vi "pigeon_ver4_1.vi"() -> ()   [LabVIEW 2015]
uses:
  <vilib>/Platform/TimedLoop/XDataNode/timing_clust.ctl
  <vilib>/Platform/TimedLoop/XDataNode/nitl_modes.ctl
  <vilib>/Platform/TimedLoop/XDataNode/wakeup.ctl
  <vilib>/rvi/Emulation/niFpgaGetClockAttributes.vi
  <vilib>/rvi/Emulation/niFpgaSctlEmulationGetInTimedLoop.vi
  <vilib>/rvi/Emulation/niFpgaEmulationReportErrorSimple.vi
  <vilib>/rvi/eio/common/nirviEmuTemplateMethod_errors.vi
  <vilib>/rvi/Emulation/niFpgaProcessEmulError.vi
  <vilib>/rvi/Emulation/niFpgaCriticalErrorInLSC.vi
  <vilib>/rvi/Memory/Memory_Emulation/nirvimemoryFastEmulation.vi
  <vilib>/rvi/Memory/Memory_Emulation/nirvimemoryEmulation.vi
  <vilib>/rvi/Emulation/niFpgaEmulationIsFPGAContextNoSignature.vi
  <vilib>/rvi/DataTransferAndStorage/Container/Common/niFpgaContainerGetUniqueNameForEmu.vi
  <vilib>/rvi/errors/nirviReportUnexpectedCaseInternalError (U32).vi
  <vilib>/rvi/interface/RandomDataEmulation/niFpgaRandomDataHandleErrors.vi
  <vilib>/eio/EIONode/EIONode.xnode
  <vilib>/Platform/TimedLoop/XDataNode/XDataNode.xnode
  <vilib>/rvi/DataTransferAndStorage/Container/XNode/niFpgaContainer.xnode
  <vilib>/rvi/interface/RandomDataEmulation/nirviRandomDataFpgaReadWriteTemplate.vi
  <vilib>/Platform/TimedLoop/XDataNode/XDNodeRunTimeDep.lvlib
panel:
  in  "AO5":i16
  out "AI2":i16
  in  "Tab Control":enum32{"pigeon"}(tab)
  out "FIFO size":i16
  in  "AO0":i16
  in  "AO1":i16
  in  "AO2":i16
  in  "Run program":bool
  in  "halt processor":bool
  out "control flags":i8 format="%b"
  in  "host operation":i16
  in  "address":u16
  in  "data1":u16
  in  "data2":i32
  in  "repeat program":i32
  out "IP address":i16
  out "PMT1":i16=-4740
  out "ReA":i32
  out "RegB":i16
  out "RegC":i16
  out "exttrigger":bool=TRUE
  out "AI1":i16=161
  out "RegD":i16
  in  "AO4":i16
  in  "AO3":i16
  out "IntTrigger":bool
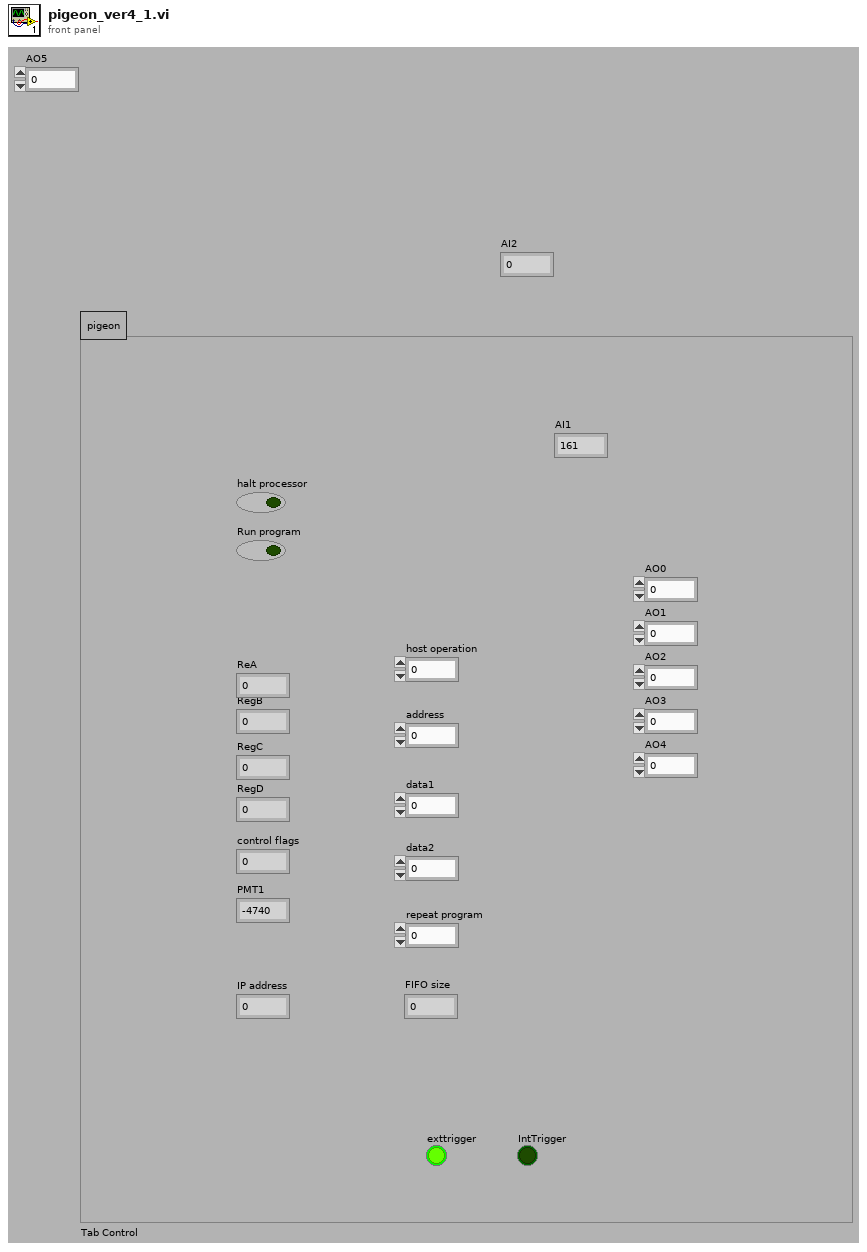
[diagram p1: front panel]
types:
  T1 = typedef "XDNodeRunTimeDep.lvlib/timing_clust.ctl" = cluster{"Expected End [f-1]":u64, "Actual End [f-1]":u64, "Finished Late? [f-1]":bool, "Expected End [i-1]":u64, "Actual End [i-1]":u64, "Finished Late? [i-1]":bool, "Expected Start [i]":u64, "Actual Start [i]":u64, "Expected Start [f]":u64, "Actual Start [f]":u64, "Source Name":string, "Structure Name":string, "Period":i64, "Deadline":i64, "Offset":i64, "Start":i64, "Priority":i32, "Timeout":i32, "Mode":T2, "Wakeup Reason":T3, "Error":errorcluster, "Source Type":string, "Secondary Source Type":string, "Global End Time":u64, "Global Start Time":u64, "Frame Duration":u64, "Iteration Duration":u64, "Assigned CPU":i32, "I/O Scan Engine Mode":u32}
  T2 = typedef "XDNodeRunTimeDep.lvlib/nitl_modes.ctl" = enum32{"No Change", "Process missed periods, maintain original phase", "Discard missed periods, maintain original phase", "Process missed periods, ignore original phase", "Discard missed periods, ignore original phase"}
  T3 = typedef "XDNodeRunTimeDep.lvlib/wakeup.ctl" = enum32{"Normal", "Aborted", "Asynchronous wakeup", "Timing source error", "Timed loop error", "Timeout"}
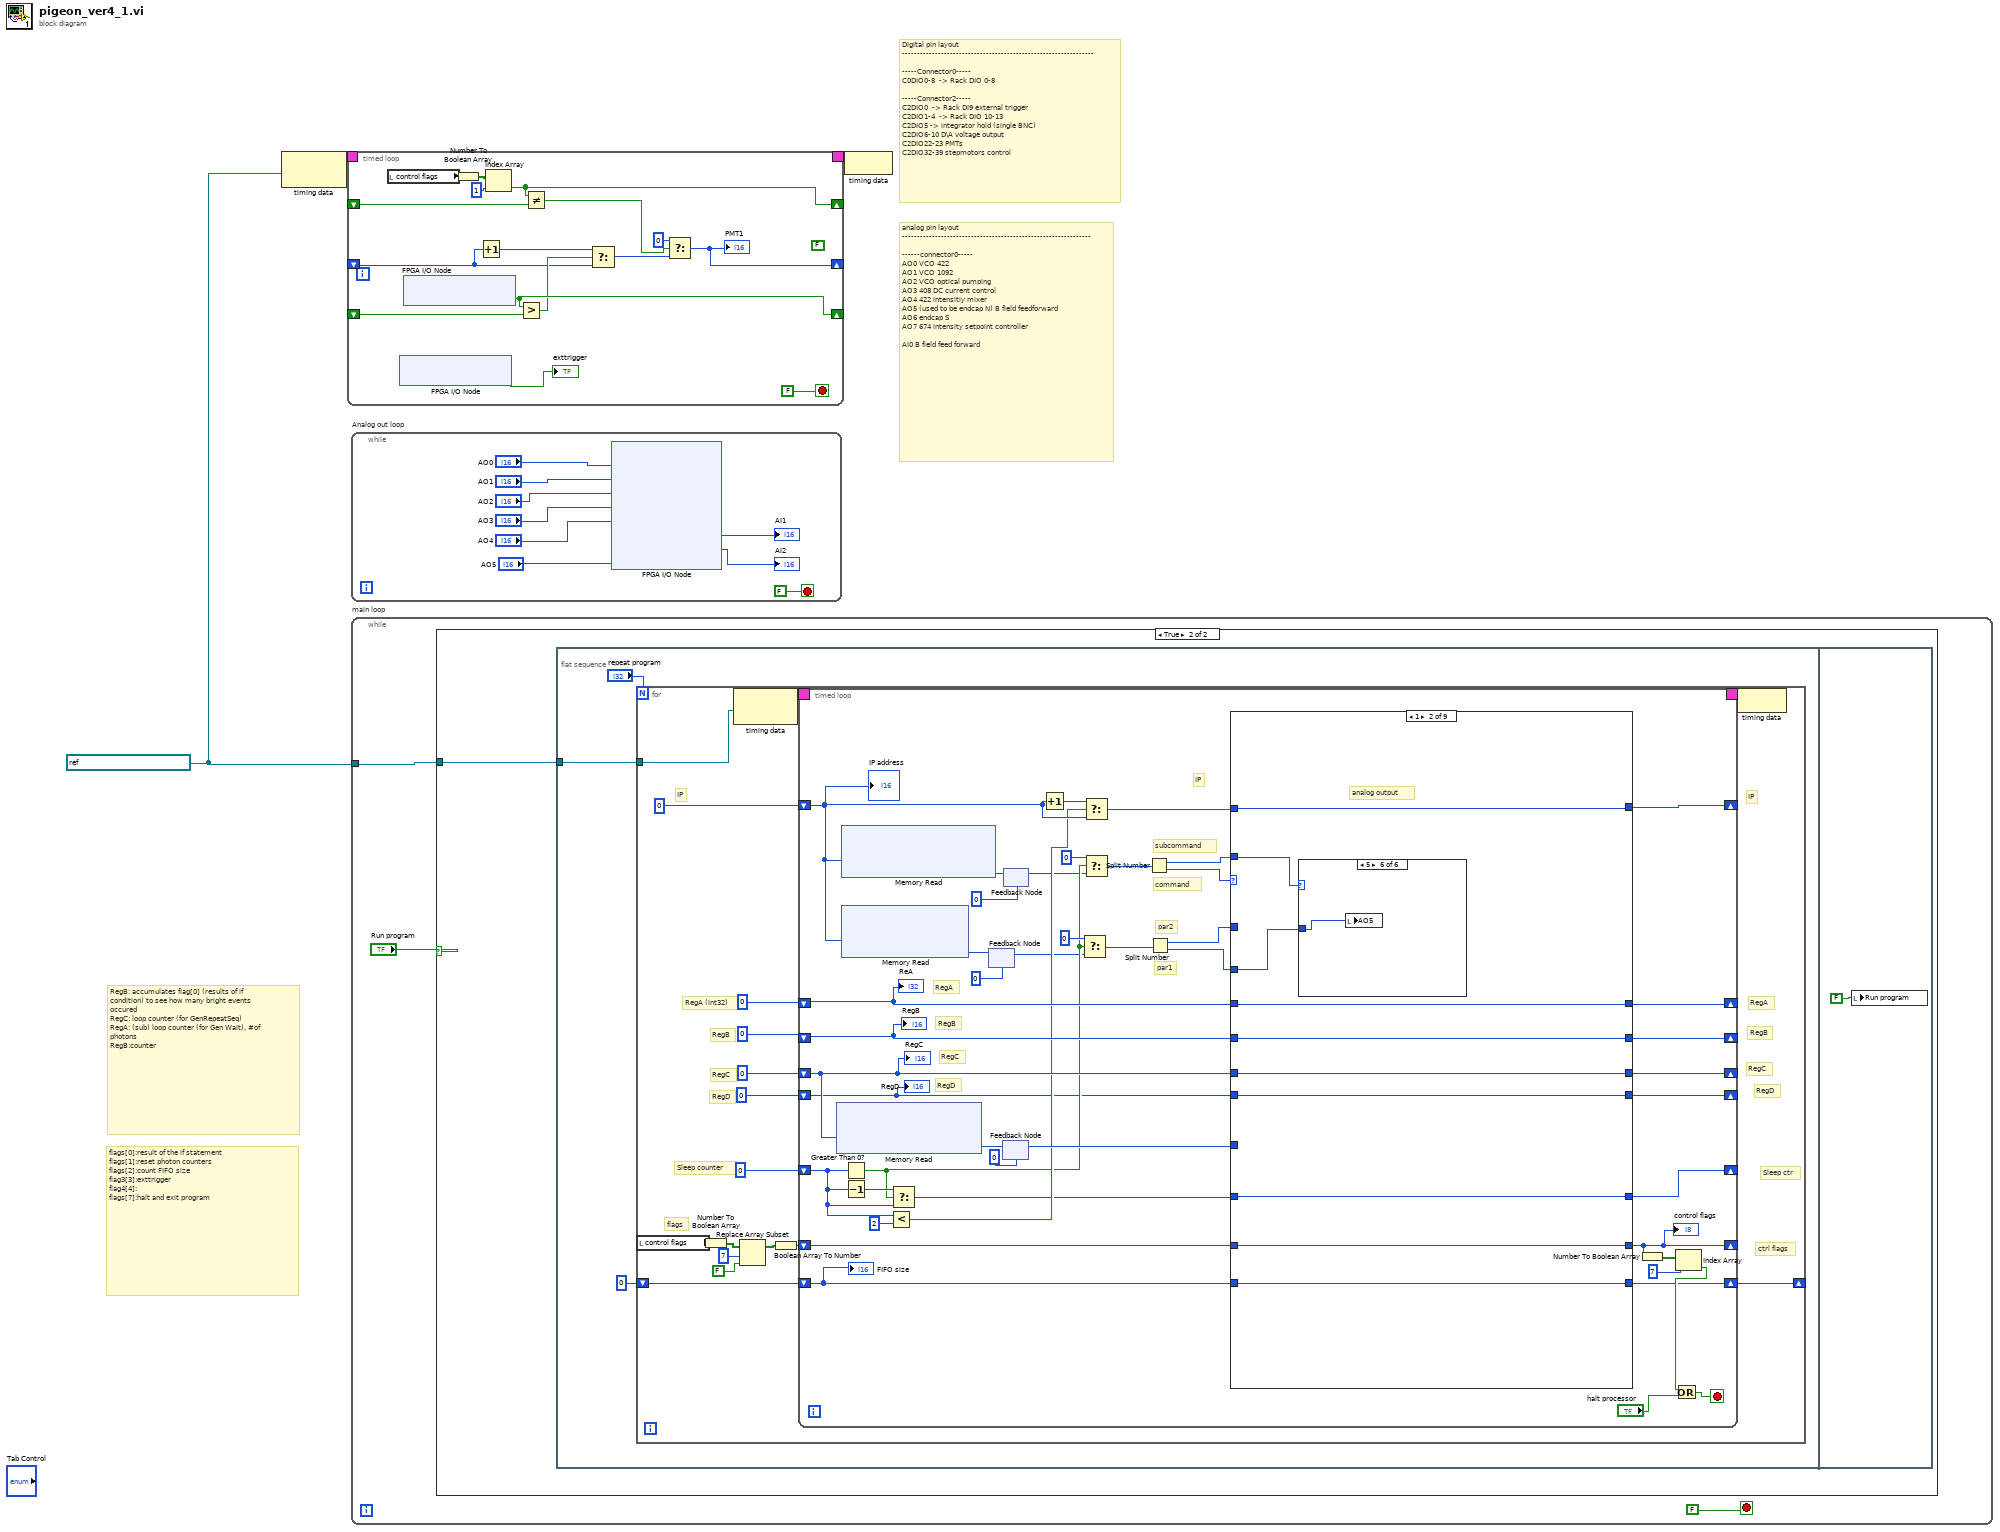
[diagram p0: block diagram]
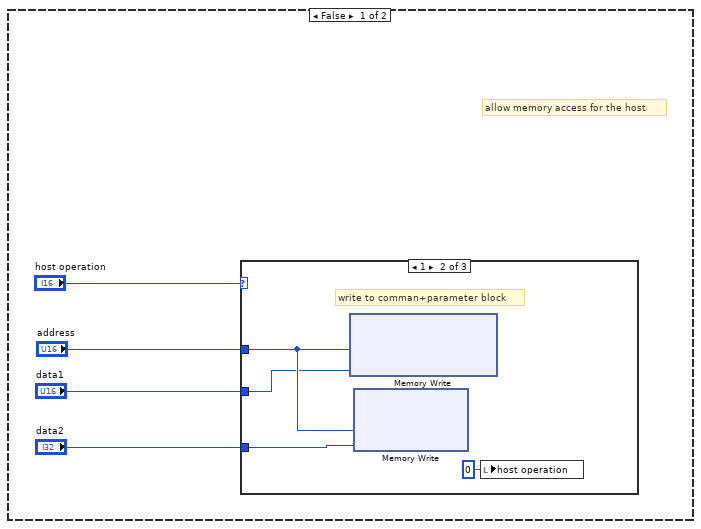
[diagram p2: hidden frame]
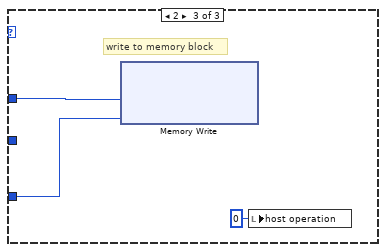
[diagram p4: hidden frame]
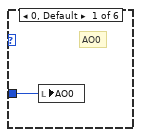
[diagram p6: hidden frame]
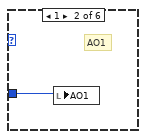
[diagram p7: hidden frame]
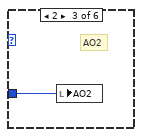
[diagram p8: hidden frame]
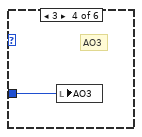
[diagram p9: hidden frame]
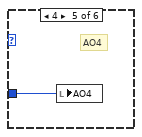
[diagram p10: hidden frame]
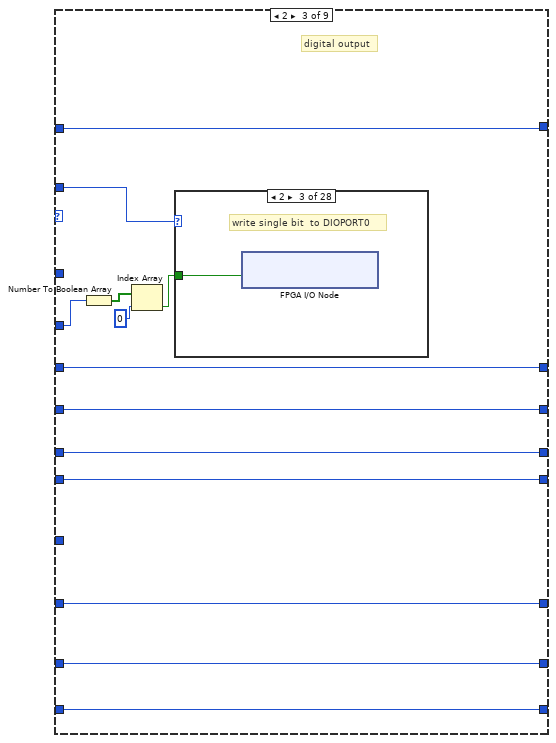
[diagram p11: hidden frame]
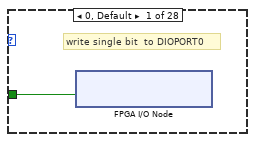
[diagram p12: hidden frame]
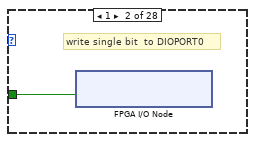
[diagram p13: hidden frame]
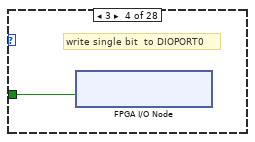
[diagram p14: hidden frame]
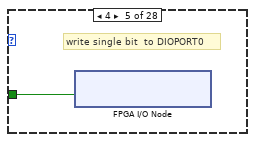
[diagram p15: hidden frame]
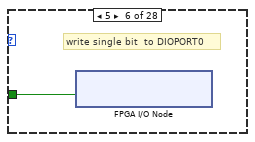
[diagram p16: hidden frame]
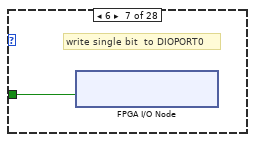
[diagram p17: hidden frame]
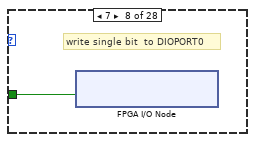
[diagram p18: hidden frame]
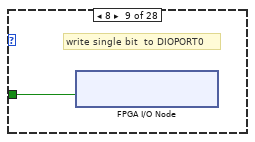
[diagram p19: hidden frame]
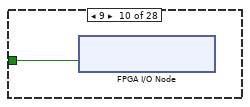
[diagram p20: hidden frame]
diagram:
  w1 = refnum<k21> "40 MHz Onboard Clock" ("FPGA Clock")
  # "RegB: accumulates flag[0] (results of if condition) to see how many bright events occured\nRegC: loop counter (for GenRepeatSeq)\nRegA: (sub) loop counter (for Gen Wait), #of     photons \nRegB:counter"
  # "flags[0]:result of the if statement\nflags[1]:reset photon counters\nflags[2]:count FIFO size\nflag3[3]:exttrigger\nflag4[4]:\nflags[7]:halt and exit program"
  # "Digital pin layout\n----------------------------------------------------------------\n\n-----Connector0-----\nC0DIO0-8  -> Rack DIO 0-8\n\n-----Connector2-----\nC2DIO0  -> Rack DI9 external trigger \nC2DIO1-4  -> Rack DIO 10-13\nC2DIO5 -> integrator hold (single BNC)\nC2DIO6-10 D\\A voltage output\nC2DIO22-23 PMTs\nC2DIO32-39 stepmotors control"
  # "analog pin layout\n---------------------------------------------------------------\n\n------connector0-----\nAO0 VCO 422\nAO1 VCO 1092\nAO2 VCO optical pumping\nAO3 408 DC current control\nAO4 422 intensitiy mixer\nAO5 (used to be endcap N) B field feedforward\nAO6 endcap S\nAO7 674 intensity setpoint controller\n\nAI0 B field feed forward"
  n1 = node-c288(w1) -> (w3:T1)
  n2 = timed-loop {
    timing: w3 -> [_]
    timing-out: [_] -> w2
    shift-right: [w17] -> _
    shift-left: _ -> [w6]
    shift-right: [w10] -> _
    shift-left: _ -> [w19]
    shift-right: [w12] -> _
    shift-left: _ -> [w13]
    stop <- FALSE stop-if-true
    (unwired) FALSE
    n3 = local read "control flags"() -> (w14:i8)
    n4 = xnode "FPGA I/O Node"() -> ("Connector2/DIO0"=→"exttrigger":bool)  [unwired: 1 in, 1 out]
    n5 = xnode "FPGA I/O Node"() -> ("Connector0/DIO0"=w10:bool)  [unwired: 1 in, 1 out]
    n6 = Number To Boolean Array(number=w14) -> (Boolean array=w15:bool[])
    n7 = Increment(x=w6) -> (x+1=w7:u16)
    n8 = Index Array(array=w15, index=1) -> (element=w12:bool)
    n9 = Greater?(x=w10, y=w19) -> (0:w9:bool)
    n10 = Not Equal?(x=w12, y=w13) -> (x != y?=w4:bool)
    n11 = Select(t=w7, s=w9, f=w6) -> (s? t:f=w18:u16)
    n12 = Select(t=u16 0, s=w4, f=w18) -> (s? t:f=w17:u16)
    "PMT1" <- w17
  }
  n13 = while "Analog out loop" {
    stop <- FALSE stop-if-true
    n14 = xnode "FPGA I/O Node"("Connector0/AO0"="AO0", "Connector0/AO1"="AO1", "Connector0/AO2"="AO2", "Connector0/AO3"="AO3", "Connector0/AO4"="AO4", "Connector0/AO5"="AO5") -> ("Connector0/AI1"=→"AI1":i16, "Connector0/AI2"=→"AI2":i16)  [unwired: 8 in, 8 out]
  }
  n15 = while "main loop" {
    tunnel: w1 -> [w31]
    stop <- FALSE ("stop") stop-if-true
    n16 = case shown="True" "Run program" {
      tunnel: w31 -> [_ w45]
      frame False {
        # "allow memory access for the host"
        n17 = case shown="1" "host operation" {
          tunnel: "address" -> [_ w39 w44]
          tunnel: "data1" -> [_ w38 _]
          tunnel: "data2" -> [_ w41 w42]
          frame 0, Default {
          }
          frame 1 {
            # "write to comman+parameter block"
            n18 = xnode ("Memory Write")("Address"=w39, "Data"=w38) -> ()  [unwired: 1 in, 1 out]
            n19 = xnode ("Memory Write")("Address"=w39, "Data"=w41) -> ()  [unwired: 1 in, 1 out]
            n20 = local write "host operation"(i16 0 ("host operation")) -> ()
          }
          frame 2 {
            # "write to memory block"
            n21 = xnode ("Memory Write")("Address"=w44, "Data"=w42) -> ()  [unwired: 1 in, 1 out]
            n22 = local write "host operation"(i16 0 ("host operation")) -> ()
          }
        }
      }
      frame True {
        n23 = flat-sequence {
          tunnel: w45 -> [w47]
          frame #0 {
            n24 = for {
              N: "repeat program" -> [_]
              tunnel: w47 -> [w59]
              shift-right: [w50] -> _
              shift-left: i16 0 -> [w51]
              # "ctrl flags"
              # "Sleep ctr"
              # "RegD"
              # "RegD"
              # "Sleep counter"
              # "flags"
              # "RegC"
              # "RegB"
              # "RegA"
              # "RegC"
              # "RegB"
              # "RegA (int32)"
              # "IP"
              # "IP"
              n25 = local read "control flags"() -> (w54:i8)
              n26 = Number To Boolean Array(number=w54) -> (Boolean array=w58:bool[])
              n27 = node-c288(w59) -> (w65:T1)
              n28 = Replace Array Subset(array=w58, new element=FALSE ("new element/subarray"), index=7) -> (w56:bool[])
              n29 = Boolean Array To Number(Boolean array=w56) -> (number=w57:u8)
              n30 = timed-loop {
                timing: w65 -> [_]
                timing-out: [_] -> w64
                shift-right: [w100] -> _
                shift-left: i16 0 -> [w83]
                shift-right: [w96] -> _
                shift-left: 0 -> [w92]
                shift-right: [w108] -> _
                shift-left: i16 0 -> [w99]
                shift-right: [w107] -> _
                shift-left: i16 0 -> [w91]
                shift-right: [w97] -> _
                shift-left: w57 -> [w98]
                shift-right: [w90] -> _
                shift-left: i16 0 -> [w81]
                shift-right: [w72] -> w50
                shift-left: w51 -> [w71]
                shift-right: [w69] -> _
                shift-left: i16 0 -> [w70]
                stop <- w103 stop-if-true
                # "RegD"
                # "IP"
                # "RegC"
                # "RegB"
                # "RegA"
                # "par1"
                # "par2"
                # "subcommand"
                # "command"
                n31 = xnode ("Memory Read")("Address"=w91) -> ("Data"=w95:i16)  [unwired: 2 in, 2 out]
                n32 = xnode ("Memory Read")("Address"=w83) -> ("Data"=w78:u16)  [unwired: 1 in, 1 out]
                n33 = xnode ("Memory Read")("Address"=w83) -> ("Data"=w74:i32)  [unwired: 1 in, 1 out]
                n34 = Greater Than 0?(x=w81) -> (x > 0?=w76:bool)
                n35 = Decrement(x=w81) -> (x-1=w82:u32)
                n36 = Less?(x=w81, y=u32 2) -> (x < y?=w80:bool)
                n37 = Select(t=w82, s=w76, f=w81) -> (s? t:f=w79:u32)
                n38 = feedback-in #1(w74) -> ()
                n39 = feedback #1(u32 0 ("Data")) -> (w73:u32)
                n40 = feedback-in #2(w95) -> ()
                n41 = feedback #2(0) -> (w94:i32)
                n42 = feedback-in #3(w78) -> ()
                n43 = feedback #3(u16 0 ("Data")) -> (w75:u16)
                n44 = Increment(x=w83) -> (x+1=w84:u16)
                n45 = Select(t=0, s=w76, f=w73) -> (s? t:f=w87:u32)
                n46 = Select(t=w84, s=w80, f=w83) -> (s? t:f=w89:u16)
                n47 = Select(t=u16 0, s=w76, f=w75) -> (s? t:f=w88:u16)
                n48 = Split Number(x=w88) -> (hi(x)=w109:u8, lo(x)=w110:u8)
                n49 = Split Number(x=w87) -> (hi(x)=w101:u16, lo(x)=w102:u16)
                n50 = case shown="1" w110 {
                  tunnel: w102 -> [_ w127 w139 _ w219 w339 w413 _ _]
                  tunnel: w101 -> [_ _ _ _ w212 w338 w412 _ _]
                  tunnel: w109 -> [_ w128 w147 w186 w220 w343 _ w431 _]
                  tunnel: w92 -> [w118 w126 w146 w178 w218 w340 w417 w435 w451]
                  tunnel: [w118 w126 w146 w178 w215 w340 w417 w435 w451] -> w96
                  tunnel: w99 -> [w117 w125 w145 w177 w217 w341 w418 w434 w454]
                  tunnel: w91 -> [w116 w124 w144 w184 w216 w342 w419 w433 w453]
                  tunnel: [w117 w125 w145 w176 w214 w341 w418 w434 w454] -> w108
                  tunnel: [w116 w124 w144 w184 w213 w342 w419 w433 w453] -> w107
                  tunnel: [w114 w123 w143 w185 w208 w346 w411 w437 w452] -> w100
                  tunnel: w89 -> [w114 w123 w143 w185 w209 w346 _ w437 w452]
                  tunnel: [w115 w122 w142 w182 w210 w345 w410 w426 w448] -> w97
                  tunnel: w98 -> [w115 w122 w142 w183 w211 w344 w410 w425 w447]
                  tunnel: w94 -> [_ _ _ _ w202 w337 _ _ _]
                  tunnel: w79 -> [w113 w121 w137 w181 w207 w336 w409 w423 w444]
                  tunnel: [w113 w121 w137 w181 w206 w336 w409 w423 w444] -> w90
                  tunnel: w71 -> [w112 w120 w136 w180 w205 w335 w408 w422 w443]
                  tunnel: [w112 w120 w136 w180 w205 w335 w408 w421 w443] -> w72
                  tunnel: w70 -> [w111 w119 w135 w179 w204 w334 w407 w420 w442]
                  tunnel: [w111 w119 w135 w179 w203 w334 w407 w420 w442] -> w69
                  frame 0, Default {
                  }
                  frame 1 {
                    # "analog output"
                    n51 = case shown="5" w128 {
                      tunnel: w127 -> [w129 w130 w131 w132 w133 w134]
                      frame 0, Default {
                        # "AO0"
                        n52 = local write "AO0"(w129) -> ()
                      }
                      frame 1 {
                        # "AO1"
                        n53 = local write "AO1"(w130) -> ()
                      }
                      frame 2 {
                        # "AO2"
                        n54 = local write "AO2"(w131) -> ()
                      }
                      frame 3 {
                        # "AO3"
                        n55 = local write "AO3"(w132) -> ()
                      }
                      frame 4 {
                        # "AO4"
                        n56 = local write "AO4"(w133) -> ()
                      }
                      frame 5 {
                        n57 = local write "AO5"(w134) -> ()
                      }
                    }
                  }
                  frame 2 {
                    # "digital output"
                    n58 = Number To Boolean Array(number=w139) -> (Boolean array=w140:bool[])
                    n59 = Index Array(array=w140, index=0) -> (element=w138:bool)
                    n60 = case shown="2" w147 {
                      tunnel: w138 -> [w148 w149 w150 w151 w152 w153 w154 w155 w156 w157 w158 w159 w160 w161 w162 w163 w164 w165 w166 w167 w168 w169 w170 w171 w172 w173 w174 w175]
                      frame 0, Default {
                        # "write single bit  to DIOPORT0"
                        n61 = xnode "FPGA I/O Node"("Connector0/DIO0"=w148) -> ()  [unwired: 1 in, 1 out]
                      }
                      frame 1 {
                        # "write single bit  to DIOPORT0"
                        n62 = xnode "FPGA I/O Node"("Connector0/DIO1"=w149) -> ()  [unwired: 1 in, 1 out]
                      }
                      frame 2 {
                        # "write single bit  to DIOPORT0"
                        n63 = xnode "FPGA I/O Node"("Connector0/DIO2"=w150) -> ()  [unwired: 1 in, 1 out]
                      }
                      frame 3 {
                        # "write single bit  to DIOPORT0"
                        n64 = xnode "FPGA I/O Node"("Connector0/DIO3"=w151) -> ()  [unwired: 1 in, 1 out]
                      }
                      frame 4 {
                        # "write single bit  to DIOPORT0"
                        n65 = xnode "FPGA I/O Node"("Connector0/DIO4"=w152) -> ()  [unwired: 1 in, 1 out]
                      }
                      frame 5 {
                        # "write single bit  to DIOPORT0"
                        n66 = xnode "FPGA I/O Node"("Connector0/DIO5"=w153) -> ()  [unwired: 1 in, 1 out]
                      }
                      frame 6 {
                        # "write single bit  to DIOPORT0"
                        n67 = xnode "FPGA I/O Node"("Connector2/DIO16"=w154) -> ()  [unwired: 1 in, 1 out]
                      }
                      frame 7 {
                        # "write single bit  to DIOPORT0"
                        n68 = xnode "FPGA I/O Node"("Connector2/DIO13"=w155) -> ()  [unwired: 1 in, 1 out]
                      }
                      frame 8 {
                        # "write single bit  to DIOPORT0"
                        n69 = xnode "FPGA I/O Node"("Connector2/DIO14"=w156) -> ()  [unwired: 1 in, 1 out]
                      }
                      frame 9 {
                        n70 = xnode "FPGA I/O Node"("Connector2/DIO1"=w157) -> ()  [unwired: 1 in, 1 out]
                      }
                      frame 10 {
                        n71 = xnode "FPGA I/O Node"("Connector2/DIO2"=w158) -> ()  [unwired: 1 in, 1 out]
                      }
                      frame 11 {
                        n72 = xnode "FPGA I/O Node"("Connector2/DIO15"=w159) -> ()  [unwired: 1 in, 1 out]
                      }
                      frame 12 {
                        n73 = xnode "FPGA I/O Node"("Connector2/DIO4"=w160) -> ()  [unwired: 1 in, 1 out]
                      }
                      frame 13 {
                        "IntTrigger" <- w161
                      }
                      frame 14 {
                        n74 = xnode "FPGA I/O Node"("Connector0/DIO6"=w162) -> ()  [unwired: 1 in, 1 out]
                      }
                      frame 15 {
                        n75 = xnode "FPGA I/O Node"("Connector0/DIO7"=w163) -> ()  [unwired: 1 in, 1 out]
                      }
                      frame 16 {
                        n76 = xnode "FPGA I/O Node"("Connector0/DIO8"=w164) -> ()  [unwired: 1 in, 1 out]
                      }
                      frame 17 {
                        n77 = xnode "FPGA I/O Node"("Connector2/DIO3"=w165) -> ()  [unwired: 1 in, 1 out]
                      }
                      frame 18 {
                        n78 = xnode "FPGA I/O Node"("Connector2/DIO18"=w166) -> ()  [unwired: 1 in, 1 out]
                      }
                      frame 19 {
                        n79 = xnode "FPGA I/O Node"("Connector2/DIO11"=w167) -> ()  [unwired: 1 in, 1 out]
                      }
                      frame 20 {
                        n80 = xnode "FPGA I/O Node"("Connector2/DIO12"=w168) -> ()  [unwired: 1 in, 1 out]
                      }
                      frame 21 {
                        n81 = xnode "FPGA I/O Node"("Connector2/DIO17"=w169) -> ()  [unwired: 1 in, 1 out]
                      }
                      frame 22 {
                        n82 = xnode "FPGA I/O Node"("Connector2/DIO19"=w170) -> ()  [unwired: 1 in, 1 out]
                      }
                      frame 23 {
                        n83 = xnode "FPGA I/O Node"("Connector2/DIO18"=w171) -> ()  [unwired: 1 in, 1 out]
                      }
                      frame 24 {
                        n84 = xnode "FPGA I/O Node"("Connector2/DIO21"=w172) -> ()  [unwired: 1 in, 1 out]
                      }
                      frame 25 {
                        n85 = xnode "FPGA I/O Node"("Connector2/DIO24"=w173) -> ()  [unwired: 1 in, 1 out]
                      }
                      frame 26 {
                        n86 = xnode "FPGA I/O Node"("Connector2/DIO25"=w174) -> ()  [unwired: 1 in, 1 out]
                      }
                      frame 27 {
                        n87 = xnode "FPGA I/O Node"("Connector2/DIO20"=w175) -> ()  [unwired: 1 in, 1 out]
                      }
                    }
                  }
                  frame 3 {
                    # "photon counting"
                    n88 = case shown="3" w186 {
                      tunnel: [w187 w189 w201] -> w176
                      tunnel: w177 -> [w187 w190 w201]
                      tunnel: w183 -> [w188 w192 w199]
                      tunnel: [w188 w192 w198] -> w182
                      frame 2, Default {
                      }
                      frame 1 {
                        # "PMT1"
                        n89 = local read "PMT1"() -> (w191:i16)
                        n90 = Add(x=w191, y=w190) -> (x+y=w189:u16)
                      }
                      frame 3 {
                        # "Reset  photon counter"
                        # "make a Not gate of flag(1)"
                        n91 = Number To Boolean Array(number=w199) -> (Boolean array=w196:bool[])
                        n92 = Index Array(array=w196, index=1) -> (element=w194:bool)
                        n93 = Not(x=w194) -> (.not. x?=w193:bool)
                        n94 = Replace Array Subset(array=w196, new element=w193, index=1) -> (w197:bool[])
                        n95 = Boolean Array To Number(Boolean array=w197) -> (number=w198:u8)
                      }
                    }
                  }
                  frame 4 {
                    # "registers operation"
                    n96 = case shown="7" w220 {
                      tunnel: w219 -> [w226 w236 w243 _ _ _ _ w285 _ _ w312 w325]
                      tunnel: w218 -> [_ w235 w242 w249 w257 w265 w269 w290 w301 w307 w317 w330]
                      tunnel: w217 -> [w229 _ w241 w248 w259 w264 w277 w289 w300 w303 w315 w328]
                      tunnel: w216 -> [w228 w234 _ w251 w258 _ w270 w288 w299 w306 w316 w329]
                      tunnel: [w225 w235 w242 w249 w256 w265 w269 w290 w301 w307 w317 w330] -> w215
                      tunnel: [w229 w236 w241 w248 w259 w264 w276 w289 w300 w305 w315 w328] -> w214
                      tunnel: [w228 w234 w243 w250 w258 w264 w270 w288 w299 w306 w316 w329] -> w213
                      tunnel: w212 -> [w227 _ _ _ _ _ _ w286 _ _ _ w324]
                      tunnel: w211 -> [w224 w233 w240 w247 w255 w263 w271 w287 w298 w310 w320 w333]
                      tunnel: [w224 w233 w240 w247 w255 w263 w271 w287 w298 w310 w320 w333] -> w210
                      tunnel: w209 -> [w223 w232 w239 w246 w254 w262 w268 w279 w293 w309 w319 w332]
                      tunnel: [w223 w232 w239 w246 w254 w262 w268 w282 w296 w309 w319 w332] -> w208
                      tunnel: w207 -> [w222 w231 w238 w245 w253 w261 w267 _ _ w308 w318 w331]
                      tunnel: [w222 w231 w238 w245 w253 w261 w267 w283 w291 w308 w318 w331] -> w206
                      tunnel: w204 -> [w221 w230 w237 w244 w252 w260 w266 w278 w292 w302 _ w323]
                      tunnel: [w221 w230 w237 w244 w252 w260 w266 w278 w292 w302 w313 w322] -> w203
                      tunnel: w202 -> [_ _ _ _ _ _ _ _ w291 _ _ _]
                      frame 0, Default {
                        # "Set par1,2 to RegA"
                        n97 = Join Numbers(hi=w227, lo=w226) -> ((hi.lo)=w225:u32)
                      }
                      frame 1 {
                        # "Set par1 to RegB"
                      }
                      frame 2 {
                        # "Set par1 to RegC"
                      }
                      frame 3 {
                        # "increase RegC by 1"
                        n98 = Increment(x=w251) -> (x+1=w250:u16)
                      }
                      frame 4 {
                        # "increase RegA by 1"
                        n99 = Increment(x=w257) -> (x+1=w256:u32)
                      }
                      frame 5 {
                        # "Set regC to regB"
                      }
                      frame 6 {
                        # "regB<-regB+flags[0]"
                        n100 = Number To Boolean Array(number=w271) -> (Boolean array=w275:bool[])
                        n101 = Index Array(array=w275, index=0) -> (element=w273:bool)
                        n102 = Boolean To (0,1)(Boolean=w273) -> (0, 1=w272:i16)
                        n103 = Add(x=w272, y=w277) -> (x+y=w276:u16)
                      }
                      frame 7 {
                        # "Sleep counter = [par1 par2]"
                        n104 = Join Numbers(hi=w286, lo=w285) -> ((hi.lo)=w283:u32)
                        n105 = Greater?(x=w283, y=u32 0) -> (0:w281:bool)
                        n106 = Decrement(x=w279) -> (x-1=w280:u16)
                        n107 = Select(t=w280, s=w281, f=w279) -> (s? t:f=w282:u16)
                      }
                      frame 11 {
                        # "Sleep counter =par1* memory Block[RegC]"
                        n108 = Greater?(x=w291, y=u32 0) -> (0:w295:bool)
                        n109 = Decrement(x=w293) -> (x-1=w294:u16)
                        n110 = Select(t=w294, s=w295, f=w293) -> (s? t:f=w296:u16)
                      }
                      frame 8 {
                        # "RegB=RegB+ RegA(lo)"
                        n111 = Split Number(x=w307) -> (lo(x)=w304:u16)  [unwired: 1 out]
                        n112 = Add(x=w304, y=w303) -> (x+y=w305:u16)
                      }
                      frame 9 {
                        # "RegD<-AI1+par1"
                        n113 = To Word Integer(number=w312) -> (16bit integer=w311:i16)
                        n114 = local read "AI1"() -> (w314:i16)
                        n115 = Add(x=w311, y=w314) -> (x+y=w313:i16)
                      }
                      frame 10 {
                        # "RegD<-RegD*2^par1*par2"
                        n116 = To Word Integer(number=w324) -> (16bit integer=w326:i16)
                        n117 = To Word Integer(number=w325) -> (16bit integer=w327:i16)
                        n118 = Multiply(x=w326, y=w323) -> (x*y=w321:i16)
                        n119 = Scale By Power Of 2(n=w327, x=w321) -> (x*2^n=w322:i16)
                      }
                    }
                  }
                  frame 5 {
                    # "If statement"
                    n120 = case shown="4" w343 {
                      tunnel: [w356 w364 w372 w380 w390 w393 w401] -> w345
                      tunnel: w344 -> [w355 w363 w371 w379 w389 w394 w402]
                      tunnel: w338 -> [w349 _ _ _ _ _ _]
                      tunnel: w342 -> [_ _ w367 w374 _ _ _]
                      tunnel: w341 -> [_ w358 _ w373 _ _ _]
                      tunnel: w340 -> [w350 _ _ _ _ w391 w399]
                      tunnel: w339 -> [w348 w357 w366 _ _ w392 _]
                      tunnel: w337 -> [_ _ _ _ _ _ w406]
                      frame 0, Default {
                        # "The if regA =  [par1,par2]"
                        n121 = Number To Boolean Array(number=w355) -> (Boolean array=w353:bool[])
                        n122 = Join Numbers(hi=w349, lo=w348) -> ((hi.lo)=w347:u32)
                        n123 = Equal?(x=w347, y=w350) -> (x = y?=w351:bool)
                        n124 = Replace Array Subset(array=w353, new element=w351, index=0) -> (w352:bool[])
                        n125 = Boolean Array To Number(Boolean array=w352) -> (number=w356:u8)
                      }
                      frame 1 {
                        # "The if  regB >  par1"
                        n126 = Number To Boolean Array(number=w363) -> (Boolean array=w361:bool[])
                        n127 = Greater?(x=w358, y=w357) -> (0:w359:bool)
                        n128 = Replace Array Subset(array=w361, new element=w359, index=0) -> (w360:bool[])
                        n129 = Boolean Array To Number(Boolean array=w360) -> (number=w364:u8)
                      }
                      frame 2 {
                        # "The if  regC=  par1"
                        n130 = Number To Boolean Array(number=w371) -> (Boolean array=w369:bool[])
                        n131 = Equal?(x=w366, y=w367) -> (x = y?=w365:bool)
                        n132 = Replace Array Subset(array=w369, new element=w365, index=0) -> (w368:bool[])
                        n133 = Boolean Array To Number(Boolean array=w368) -> (number=w372:u8)
                      }
                      frame 3 {
                        # "The if  regB> regC"
                        n134 = Number To Boolean Array(number=w379) -> (Boolean array=w377:bool[])
                        n135 = Greater?(x=w373, y=w374) -> (0:w375:bool)
                        n136 = Replace Array Subset(array=w377, new element=w375, index=0) -> (w376:bool[])
                        n137 = Boolean Array To Number(Boolean array=w376) -> (number=w380:u8)
                      }
                      frame 4 {
                        w385 = 3 ("index")
                        # "external trigger rising edge"
                        n138 = Number To Boolean Array(number=w389) -> (Boolean array=w386:bool[])
                        n139 = local read "exttrigger"() -> (w382:bool)
                        n140 = Index Array(array=w386, index=w385) -> (element=w384:bool)
                        n141 = Not(x=w384) -> (.not. x?=w383:bool)
                        n142 = And(x=w382, y=w383) -> (x .and. y?=w381:bool)
                        n143 = Replace Array Subset(array=w386, new element #1=w381, index #1=0 ("index"), new element #2=w382, index #2=w385) -> (w387:bool[])
                        n144 = Boolean Array To Number(Boolean array=w387) -> (number=w390:u8)
                      }
                      frame 5 {
                        # "The if  regA >  par1"
                        n145 = Number To Boolean Array(number=w394) -> (Boolean array=w397:bool[])
                        n146 = Greater?(x=w391, y=w392) -> (0:w395:bool)
                        n147 = Replace Array Subset(array=w397, new element=w395, index=0) -> (w396:bool[])
                        n148 = Boolean Array To Number(Boolean array=w396) -> (number=w393:u8)
                      }
                      frame 6 {
                        # "The if  regA == memoryBlock(regC)"
                        n149 = Number To Boolean Array(number=w402) -> (Boolean array=w404:bool[])
                        n150 = Equal?(x=w399, y=w406) -> (x = y?=w400:bool)
                        n151 = Replace Array Subset(array=w404, new element=w400, index=0) -> (w403:bool[])
                        n152 = Boolean Array To Number(Boolean array=w403) -> (number=w401:u8)
                      }
                    }
                  }
                  frame 6 {
                    # "condition (flags[0]) goto\nuse par1=par2 for normal goto"
                    n153 = Number To Boolean Array(number=w410) -> (Boolean array=w416:bool[])
                    n154 = Index Array(array=w416, index=0) -> (element=w414:bool)
                    n155 = Select(t=w413, s=w414, f=w412) -> (s? t:f=w411:u16)
                  }
                  frame 7 {
                    w424 = 2 ("index")
                    # "make a Not gate of flag(2)"
                    # "push  to FIFO"
                    n156 = case shown="0, Default" w431 {
                      tunnel: w435 -> [w438 _ _ _]
                      tunnel: w434 -> [_ w439 _ _]
                      tunnel: w433 -> [_ _ w440 _]
                      tunnel: [w438 w439 w440 w441] -> w432
                      frame 0, Default {
                        # "push RegA"
                      }
                      frame 1 {
                        # "push RegB"
                      }
                      frame 2 {
                        # "push RegC"
                      }
                      frame 4 {
                        n157 = local read "AI1"() -> (w441:i16)
                      }
                    }
                    n158 = Number To Boolean Array(number=w425) -> (Boolean array=w429:bool[])
                    n159 = Index Array(array=w429, index=w424) -> (element=w428:bool)
                    n160 = Not(x=w428) -> (.not. x?=w427:bool)
                    n161 = Replace Array Subset(array=w429, new element=w427, index=w424) -> (w430:bool[])
                    n162 = Increment(x=w422) -> (x+1=w421:i16)
                    n163 = xnode ("FIFO Write")("Element"=w432, "Timeout"=0) -> ()  [unwired: 1 in, 2 out]
                    n164 = Boolean Array To Number(Boolean array=w430) -> (number=w426:u8)
                  }
                  frame 8 {
                    # "Stop and reset program"
                    n165 = Number To Boolean Array(number=w447) -> (Boolean array=w450:bool[])
                    n166 = Replace Array Subset(array=w450, new element=TRUE ("new element/subarray"), index=7) -> (w449:bool[])
                    n167 = Boolean Array To Number(Boolean array=w449) -> (number=w448:u8)
                  }
                }
                "control flags" <- w97
                n168 = Number To Boolean Array(number=w97) -> (Boolean array=w106:bool[])
                n169 = Index Array(array=w106, index=7) -> (element=w104:bool)
                n170 = Or(x=w104, y="halt processor") -> (x .or. y?=w103:bool)
                "IP address" <- w83
                "ReA" <- w92
                "RegB" <- w99
                "RegC" <- w91
                "FIFO size" <- w71
                "RegD" <- w70
              }
              n171 = node-c288(w64) -> ()
            }
          }
          frame #1 {
            n172 = local write "Run program"(FALSE ("Run program")) -> ()
          }
        }
      }
    }
  }
  n173 = node-c288(w2) -> ()
